vi "循环计数.vi"(11 "0-最大值":u8=15) -> (3 "循环计数":u8)   [LabVIEW 2020]
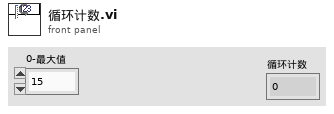
[diagram p1: front panel]
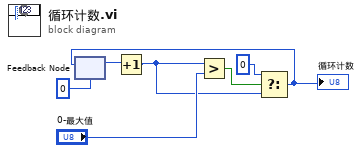
[diagram p0: block diagram]
diagram:
  n1 = feedback #1(u8 0) -> (w7:u8)
  n2 = Increment(x=w7) -> (x+1=w3:u8)
  n3 = Greater?(x=w3, y="0-最大值") -> (0:w4:bool)
  n4 = Select(t=u8 0, s=w4, f=w3) -> (s? t:f=w2:u8)
  "循环计数" <- w2
  n5 = feedback-in #1(w2) -> ()
